vi "New Light.vi"(8 "error in (no error)":errorcluster, 10 "Light Number":i32, 11 "At Infinity":bool) -> (0 "error out":errorcluster, 3 "New Light Refnum":refnum<vi>)   [LabVIEW 2017, in "NI_3D Picture Control.lvlib"]
doc: "Creates a new light source for the 3D scene."
uses:
  <vilib>/picture/3D Picture Control/NI_3D Picture Control.lvlib
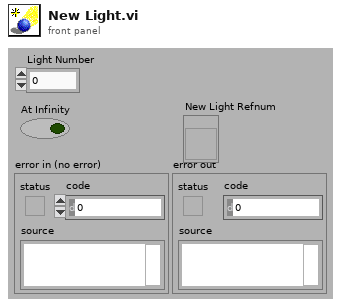
[diagram p1: front panel]
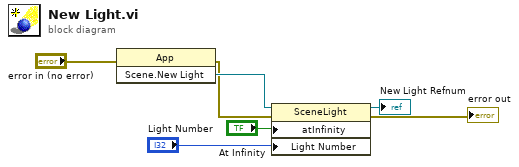
[diagram p0: block diagram]
diagram:
  n1 = invoke class="App" method="Scene.New Light"(error in="error in (no error)") -> (error out=w6:errorcluster, "Scene.New Light"=w7:refnum<vi>)  [unwired: 2 in, 1 out]
  n2 = property class="SceneLight"(reference=w7, error in=w6, "atInfinity"="At Infinity", "Light Number"="Light Number") -> (reference out=→"New Light Refnum":refnum<vi>, error out=→"error out":errorcluster)
